vi "Save Data Process.vi"(8 "error in (no error)":errorcluster, 10 "Fiber Auto Collimation state data in":refnum<class "Fiber Auto Collimation state data.lvclass">, 11 "Station config in":refnum<class "Station config.lvclass">) -> (0 "error out":errorcluster, 2 "Fiber Auto Collimation state data out":refnum<class "Fiber Auto Collimation state data.lvclass">, 3 "Station config out":refnum<class "Station config.lvclass">)   [LabVIEW 2018]
uses:
  State data/Fiber Auto Collimation state data.lvclass
  <userlib>/Recipe/Station Config/Station config.lvclass
  <userlib>/nLight Tidbits/Logging/Controls/Logging type choice.ctl
  <instrlib>/nLight Instruments/Motion Controller/Axis index.ctl
  <instrlib>/nLight Instruments/Motion Controller/Motion Controller.lvclass
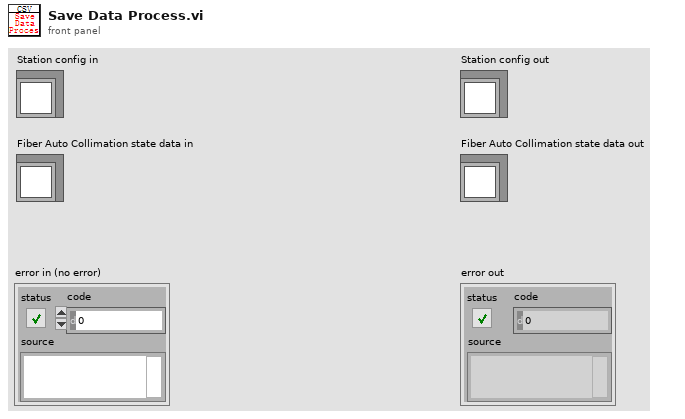
[diagram p1: front panel]
types:
  T1 = typedef "Logging type choice.ctl" = enum16{"No log type selected", "Testing start/stop", "Test progress", "Station startup/shutdown", "Station config change", "Recipe load/change", "Inventory transaction", "Instrument", "Debug"}
  T2 = typedef "Motion Controller.lvclass/Axis index.ctl" = i32
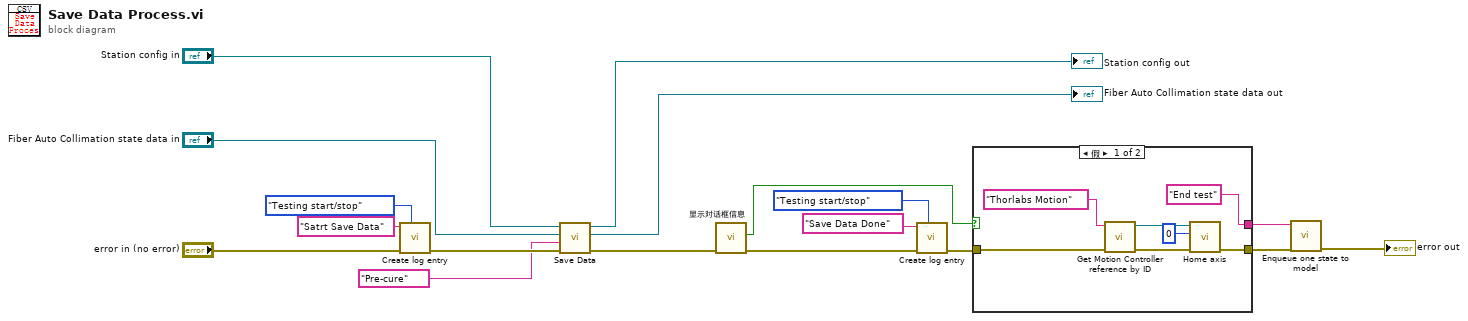
[diagram p0: block diagram]
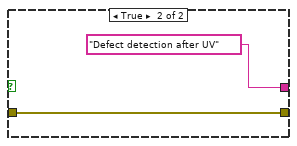
[diagram p2: hidden frame]
diagram:
  n1 = call <userlib>:"Create log entry.vi"("Logging type choice"=Logging_type_choice."Testing start/stop", "error in (no error)"="error in (no error)", "Brief log entry"="Satrt Save Data") -> ("error out"=w14:errorcluster)  [unwired: 8 in]
  n2 = call "Save Data.vi"("error in (no error)"=w14, "Process Sub Step"="Pre-cure", "Fiber Auto Collimation state data in"="Fiber Auto Collimation state data in", "Station config in"="Station config in") -> ("error out"=w7:errorcluster, "Fiber Auto Collimation state data out"=→"Fiber Auto Collimation state data out":refnum<class "Fiber Auto Collimation state data.lvclass">, "Station config out"=→"Station config out":refnum<class "Station config.lvclass">)  [unwired: 5 in]
  n3 = call "显示对话框信息"("error in (no error)"=w7) -> ("error out"=w6:errorcluster, "确定"=w3:bool)  [unwired: 9 in]
  n4 = call <userlib>:"Create log entry.vi"("Logging type choice"=Logging_type_choice."Testing start/stop", "error in (no error)"=w6, "Brief log entry"="Save Data Done") -> ("error out"=w5:errorcluster)  [unwired: 8 in]
  n5 = case shown="假" w3 {
    tunnel: w5 -> [w22 w27]
    tunnel: [w24 w27] -> w4
    tunnel: ["End test" ("Enqueued state") "Defect detection after UV" ("Enqueued state")] -> w2
    frame False {
      n6 = call <instrlib>:"Get Motion Controller reference by ID.vi"("error in (no error)"=w22, "Identifier"="Thorlabs Motion") -> ("error out"=w21:errorcluster, "Motion Controller out"=w20:refnum<class "Motion Controller.lvclass">)  [unwired: 8 in]
      n7 = call-dynamic "Home axis.vi"("error in (no error)"=w21, "Axis index"=T2 0, "Motion Controller in"=w20) -> ("error out"=w24:errorcluster)  [unwired: 7 in, 1 out]
    }
    frame True {
    }
  }
  n8 = call "Enqueue one state to model.vi"("error in (no error)"=w4, "Enqueued state"=w2) -> ("error out"=→"error out":errorcluster)  [unwired: 9 in]
